vi "test--load all the images in a directory.vi"() -> ()   [LabVIEW 2021]
panel:
  in  "File Path":path
  out "Array - Numeric":i32[](array[numeric])
  out "size(s)":i32
  out "Array":cluster{"2D Picture":picture, "path":path}[][](array[cluster])
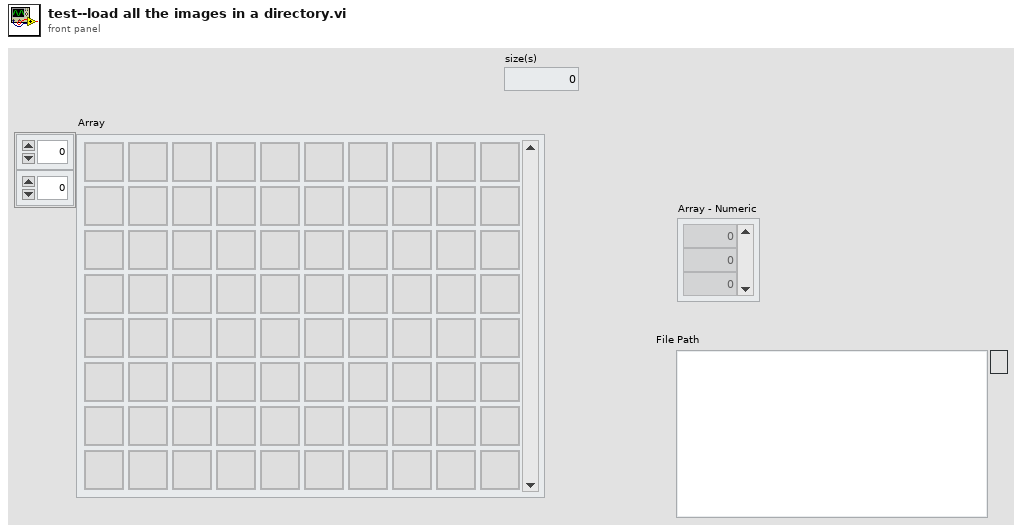
[diagram p1: front panel]
types:
  T1 = typedef "imagedata.ctl" = cluster{"image type":i32, "image depth":i32, "image":u8[], "mask":u8[], "colors":u32[], "Rectangle":cluster{"left":i16, "top":i16, "right":i16, "bottom":i16}}
  T2 = typedef "LVPoint32TypeDef.ctl" = cluster{"Horizontal":i32, "Vertical":i32}
  T3 = cluster{"data name":string, "drag data":variant}[]
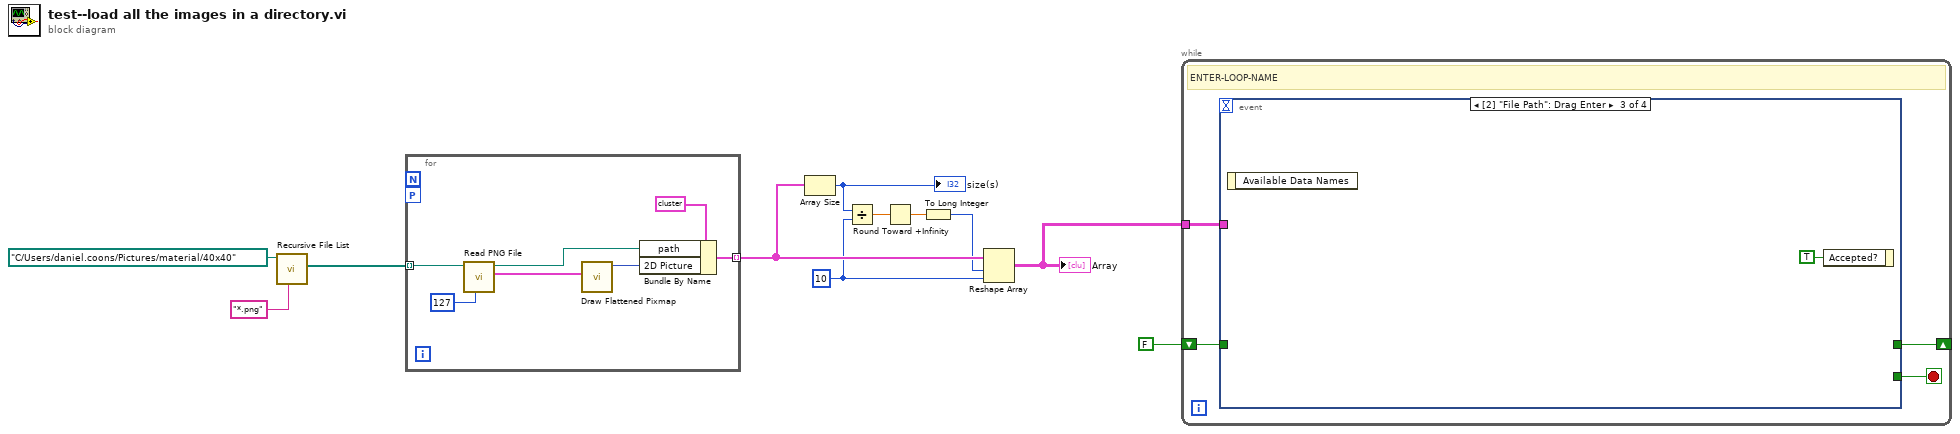
[diagram p0: block diagram]
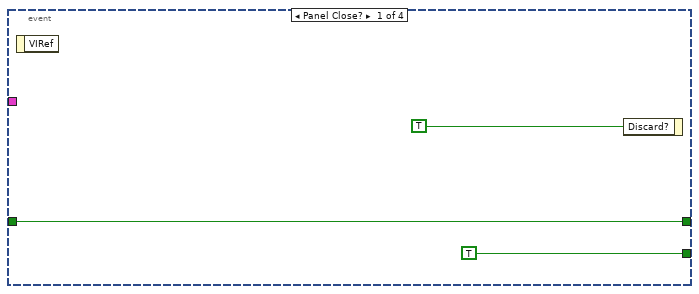
[diagram p2: hidden frame]
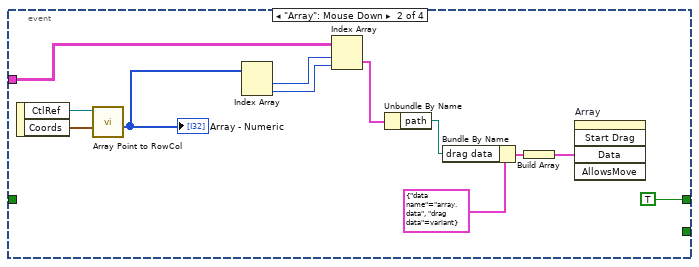
[diagram p3: hidden frame]
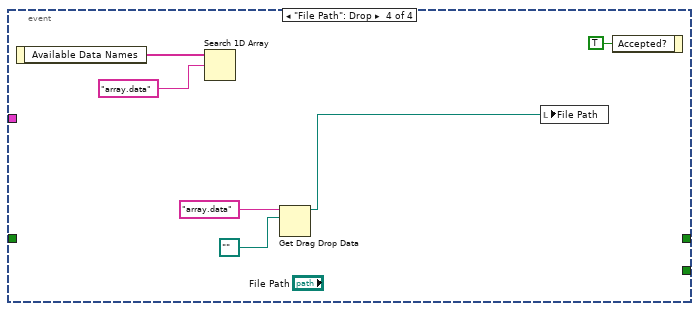
[diagram p4: hidden frame]
diagram:
  w4 = 10 ("dimension size")
  n1 = call <vilib>:"Recursive File List.vi"("pattern"="*.png", "Folder Path"=path "C:/Users/daniel.coons/Pictures/material/40x40") -> ("All Files in Dir"=w3:path[])  [unwired: 5 in, 4 out]
  n2 = for {
    tunnel: w3 -> [w18] mode=indexing
    tunnel: [w16] -> w9 mode=indexing
    workers-P: _ -> [_]
    n3 = call <vilib>:"Read PNG File.vi"("Transparency Thresh"=u8 127, "path to PNG file"=w18) -> ("image data"=w17:T1, "path"=w12:path)  [unwired: 7 in, 1 out]
    n4 = call <vilib>:"Draw Flattened Pixmap.vi"("image data"=w17) -> ("new picture"=w13:picture)  [unwired: 8 in]
    n5 = Bundle By Name(cluster=cluster{"2D Picture":picture, "path":path} {"2D Picture"=bytes[0], "path"=path ""} ("Cluster"), "path"=w12, "2D Picture"=w13) -> (w16:cluster{"2D Picture":picture, "path":path})
  }
  n6 = Array Size(array=w9) -> (size(s)=w8:i32)
  "size(s)" <- w8
  n7 = Divide(x=w8, y=w4) -> (x/y=w7:dbl)
  n8 = Round Toward +Infinity(x=w7) -> (ceil(x): smallest int >= x=w6:dbl)
  n9 = To Long Integer(number=w6) -> (32bit integer=w5:i32)
  n10 = Reshape Array(w9, w5, w4) -> (w2:cluster{"2D Picture":picture, "path":path}[][])
  "Array" <- w2
  n11 = while {
    tunnel: w2 -> [w21]
    shift-right: [w19] -> _
    shift-left: FALSE -> [w20]
    stop <- w22 stop-if-true
    # "ENTER-LOOP-NAME"
    n12 = event shown="[2] \"File Path\": Drag Enter" {
      selector: _ -> [_ _ _ _]
      dyn-events: _ -> [_ _ _ _]
      timeout: _ -> [_ _ _ _]
      tunnel: [TRUE _ _ _] -> w22
      tunnel: w21 -> [_ w34 _ _]
      tunnel: w20 -> [w23 _ _ _]
      tunnel: [w23 TRUE _ _] -> w19
      event Panel Close? {
        n13 = event-data() -> ()  [unwired: 1 in, 1 out]
        n14 = event-data("Discard?"=TRUE) -> ()  [unwired: 1 in, 1 out]
      }
      event "Array": Mouse Down {
        n15 = event-data() -> ("CtlRef"=w37:refnum<vi>, "Coords"=w36:T2)  [unwired: 1 in]
        n16 = call "Array Point to RowCol.vi"("Mouse Coords"=w36, "Array Ref"=w37) -> ("Clicked Index"=w33:i32[])  [unwired: 6 in, 3 out]
        "Array - Numeric" <- w33
        n17 = Index Array(array=w33) -> (element #1=w32:i32, element #2=w31:i32)  [unwired: 2 in]
        n18 = Index Array(array=w34, index (row)=w32, index (col)=w31) -> (element=w30:cluster{"2D Picture":picture, "path":path})
        n19 = Unbundle By Name(w30) -> ("path"=w27:path)
        n20 = Bundle By Name(cluster=cluster{"data name":string, "drag data":variant} {"data name"="array.data", "drag data"=variant}, "drag data"=w27) -> (w28:cluster{"data name":string, "drag data":variant})
        n21 = Build Array(w28) -> (w26:T3)
        n22 = invoke on="Array" class="Arr (strict)" method="Start Drag"("Data"=w26) -> ()  [unwired: 4 in, 5 out]
      }
      event "File Path": Drag Enter {
        n23 = event-data() -> ()  [unwired: 1 in, 1 out]
        n24 = event-data("Accepted?"=TRUE) -> ()  [unwired: 1 in, 1 out]
      }
      event "File Path": Drop {
        n25 = event-data() -> ("Available Data Names"=w43:string[])  [unwired: 1 in]
        n26 = Search 1D Array(1D array=w43, element="array.data") -> ()  [unwired: 1 in, 1 out]
        n27 = Get Drag Drop Data(8:path "", 9:"array.data" ("data name")) -> (3:w39:path)  [unwired: 1 in, 1 out]
        n28 = local write "File Path"(w39) -> ()
        n29 = event-data("Accepted?"=TRUE) -> ()  [unwired: 1 in, 1 out]
      }
    }
  }
